vi "Translator.File.Read.Msg.vi"(4 "progressbar2":refnum<vi>, 6 "progressbar1":refnum<vi>, 7 "Message":refnum<vi>, 8 "error in":errorcluster, 11 "Translation folder":path=path "D:/PL_0125_Sapphire_Automation_branches/SOFTWARE_v1.1-Translation/settings/Translation-Chinese.ini") -> (0 "error out":errorcluster)   [LabVIEW 2016]
uses:
  Translator.Enums.ctl
  Translator.Message.ctl
  EventLog/EventLog.EventLevelGui.ctl
  Windows/Windows.ExitAction.ctl
  TouchPanel/TouchPanelMonths.ctl
  EventLog/EventLog.EventSource.ctl
  Translator.File.MatchStrings (Array).vi
  <vilib>/Utility/config.llb/NI_LVConfig.lvlib
panel:
  out "#old":i32[](array[numeric])
  out "#new":i32[](array[numeric])
  in  "Enums":T1={"Msg"=enum."Quitting", "Level"=enum."ALL", "ExitAction"=enum."Log off from PC", "Month"=enum."January", "Source"=enum."Gui"}
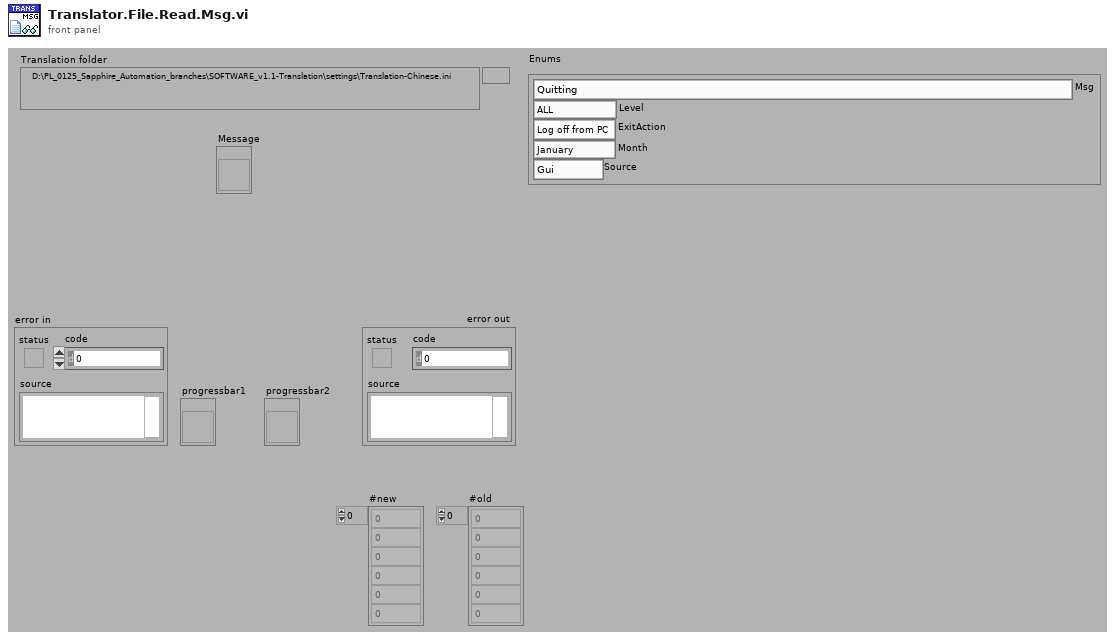
[diagram p1: front panel]
types:
  T1 = typedef "Translator.Enums.ctl" = cluster{"Msg":T2, "Level":T3, "ExitAction":T4, "Month":T5, "Source":T6}
  T2 = typedef "Translator.Message.ctl" = enum16{"-", "Event confirmed", "Log out", "Log in", "Shutdown", "Cancel", "Start", "Continue", "Stop", "On", "Off", "OK", "NOK", "NOK %s", "This", "Prev", "Home", "Work", "In progress...", "Missing", "Empty", "Hardware failure", "Initial", "Error %d >> %s", "Error %d >> %s >> %s", "Starting %s", "Quitting %s", "Configured", "Initializing", "Quitting", "Loading", "Running %s", "Stopped", "Summary", "Do you want to continue?", "Do you want to exit?", "Log out?", "System", "All", "IDLE", "Translating...%s", "Not found", "Alarm %s", "Run", "Skip", "Abort", "Repeat", "Please wait...", "Database disconnected", "Login to database successful", "Login to database failed: %d; %s", "Get process step data for %s", "Changeover off", "Changeover into %s", "Product %s | %s found in cache with status %d at previous station", "Product %s | %s found in database with status %d at previous station", "Product %s | %s not found in cache at previous station", "Product %s | %s not found in database at previous station", "Product %s | %s found in cache with status %d at this station (%d repetion)", "Product %s | %s found in database with status %d at this station (%d repetition)", "Product %s | %s not found in cache at this station", "Product %s | %s not found in database at this station", "Product %s | %s found in cache for component %s | %s", "Product %s | %s found in database for component %s | %s", "Product not found in cache for component %s | %s", "Product not found in database for component %s | %s", "Product %s | %s connected with component %s | %s (cache)", "Product %s | %s connected with component %s | %s (database)", "New data for %s | %s (cache)", "New data for %s | %s (database)", "File %s moved (cache)", "File %s deleted (cache)", "Msg %d >> %s", "PLC LifeBit Failure", "Reconnecting DB", "Reconnecting PLC", "Free disk space is below 1GB - contact technician", "Unable to check product status", "Product %s SN %s checked in DB", "Unable To check status from station %s"}
  T3 = typedef "EventLog.EventLevelGui.ctl" = enum16{"ALL", "Debug", "Info", "Warning", "Error"}
  T4 = typedef "Windows.ExitAction.ctl" = enum16{"Log off from PC", "Shut Down PC", "Reboot PC", "Close Program"}
  T5 = typedef "TouchPanelMonths.ctl" = enum16{"January", "February", "March", "April", "May", "June", "July", "August", "September", "October", "November", "December"}
  T6 = typedef "EventLog.EventSource.ctl" = enum16{"All", "Gui", "Cache", "PLC1", "PLC2", "PLC3", "DB", "DB01", "DB02", "DB03", "DB04", "DB05", "DB06", "DB07", "DB08", "DB09", "DB10", "DB11", "DB12", "DB13", "DB14", "DB15", "DB16"}
  T7 = typedef "NI_LVConfig.lvlib/Config Data RefNum.ctl" = refnum<k1>
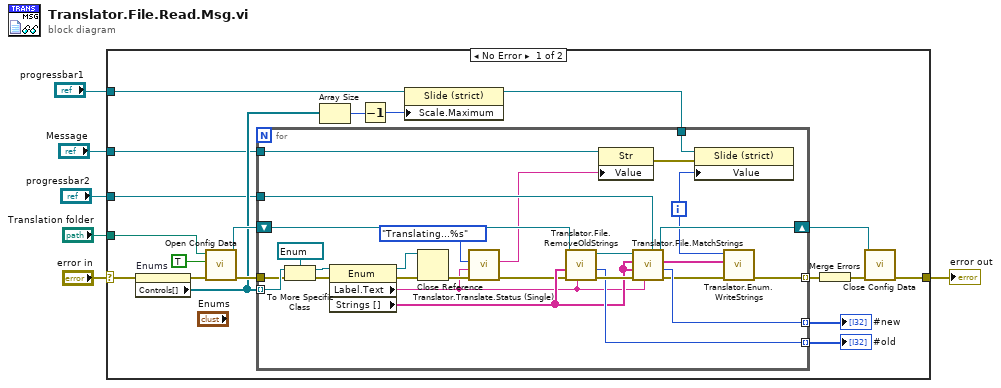
[diagram p0: block diagram]
diagram:
  n1 = case shown="No Error" "error in" {
    selector: "error in" -> [w21 w53]
    tunnel: "Translation folder" -> [w18 _]
    tunnel: [w19 w53] -> w5
    tunnel: "progressbar1" -> [w11 _]
    tunnel: "progressbar2" -> [w10 _]
    tunnel: "Message" -> [w8 _]
    frame No Error {
      n2 = property on="Enums" class="Clust (strict)"(error in=w21) -> (error out=w20:errorcluster, "Controls[]"=w12:refnum<vi>[])  [unwired: 1 in, 1 out]
      n3 = call <vilib>:"Open Config Data.vi"("error in (no error)"=w20, "create file if necessary (T)"=TRUE, "configuration file path"=w18) -> ("error out"=w23:errorcluster, "refnum"=w16:T7)  [unwired: 6 in, 1 out]
      n4 = Array Size(array=w12) -> (size(s)=w13:i32)
      n5 = Decrement(x=w13) -> (x-1=w14:i32)
      n6 = property on="Property Node" class="Slide (strict)"(reference=w11, "Scale.Maximum"=w14) -> (reference out=w9:refnum<vi>)  [unwired: 1 in, 1 out]
      n7 = for {
        tunnel: w12 -> [w52] mode=indexing
        shift-right: [w41] -> w15
        shift-left: w16 -> [w45]
        tunnel: [w40] -> w22 mode=indexing
        tunnel: [w42] -> w17 mode=indexing
        tunnel: w10 -> [w37]
        tunnel: w9 -> [w38]
        tunnel: w8 -> [w36]
        tunnel: w23 -> [w48]
        tunnel: [w26] -> w24 mode=indexing
        i -> [w27]
        n8 = To More Specific Class(target class=refnum<vi> refnum ("reference out"), reference=w52, error in=w48) -> (specific class reference=w51:refnum<vi>, error out=w50:errorcluster)
        n9 = property class="Enum"(reference=w51, error in=w50) -> (reference out=w46:refnum<vi>, error out=w47:errorcluster, "Label.Text"=w30:string, "Strings []"=w39:string[])
        n10 = Close Reference(reference=w46, error in (no error)=w47) -> (error out=w34:errorcluster)
        n11 = call "Translator.Translate.Status (Single).vi"("error in (no error)"=w34, "Arg"=w30, "Msg"=Translator.Message."Translating...%s" ("msg")) -> ("error out"=w33:errorcluster, "Translated Msg"=w31:string)  [unwired: 7 in]
        n12 = call "Translator.File.RemoveOldStrings.vi"("group"=w30, "error in"=w33, "labels"=w39, "refnum in"=w45) -> ("error out"=w44:errorcluster, "#removed"=w42:i32, "refnum out"=w43:T7)  [unwired: 5 in]
        n13 = property on="Property Node" class="Str"(reference=w36, "Value"=w31) -> (error out=w35:errorcluster)  [unwired: 1 in, 1 out]
        n14 = call-poly "Translator.File.MatchStrings.vi"("progressbar"=w37, "group"=w30, "error in"=w44, "labels"=w39, "default values"=w39, "refnum in"=w43) -> ("error out"=w29:errorcluster, "#added"=w40:i32, "values out"=w28:string[], "refnum out"=w41:T7)  [unwired: 2 in]
        n15 = property on="Property Node" class="Slide (strict)"(reference=w38, error in=w35, "Value"=w27) -> ()  [unwired: 2 out]
        n16 = call "Translator.Enum.WriteStrings.vi"("error out"=w29, "Strings"=w28, "idx"=w27) -> ("error out 2"=w26:errorcluster)  [unwired: 8 in]
      }
      "#new" <- w22
      "#old" <- w17
      n17 = Merge Errors(w24) -> (w7:errorcluster)
      n18 = call <vilib>:"Close Config Data.vi"("error in (no error)"=w7, "refnum"=w15) -> ("error out"=w19:errorcluster)  [unwired: 8 in, 1 out]
    }
    frame Error {
    }
  }
  "error out" <- w5
